vi "AI mnoz wartosci analogowe.vi"(6 "Mnozniki in":dbl[](array[numeric]), 7 "#cores (1)":i32=1, 8 "error in (no error)":errorcluster, 10 "Kanaly in":T1) -> (0 "error out":errorcluster, 2 "Kanaly out":T1, 5 "Niezgodnosc rozmiarow?":bool)   [LabVIEW 2013]
doc: "Mnoży wartości na aktywnych kanałach analogowych\nprzez mnożniki wyliczone z ustawien kart analogowych przystawki"
uses:
  Kontrolki/Przetwarzanie/Kanaly.ctl
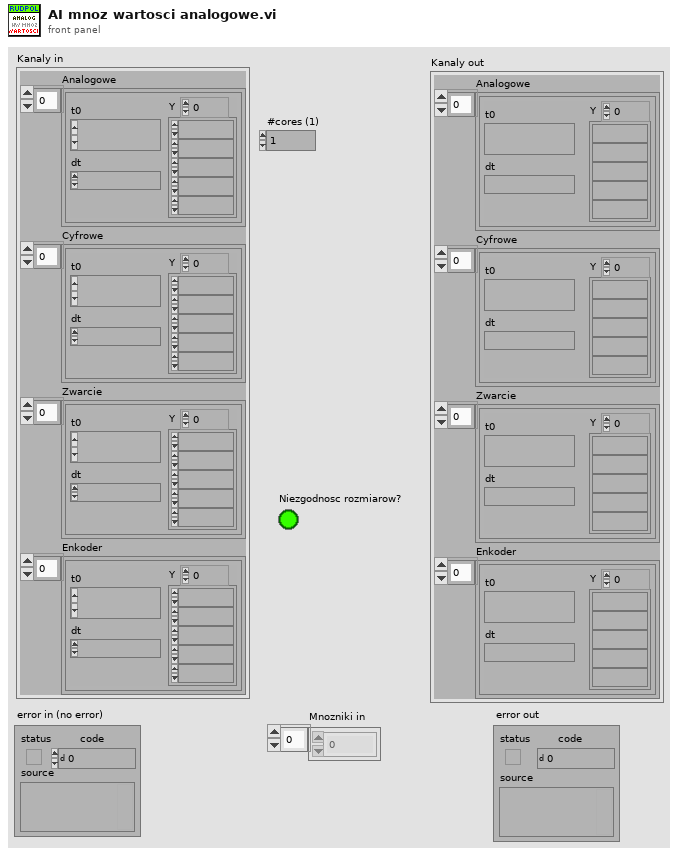
[diagram p1: front panel]
types:
  T1 = typedef "Kanaly.ctl" = cluster{"Analogowe":waveform(dbl)[], "Cyfrowe":waveform(dbl)[], "Zwarcie":waveform(dbl)[], "Enkoder":waveform(dbl)[]}
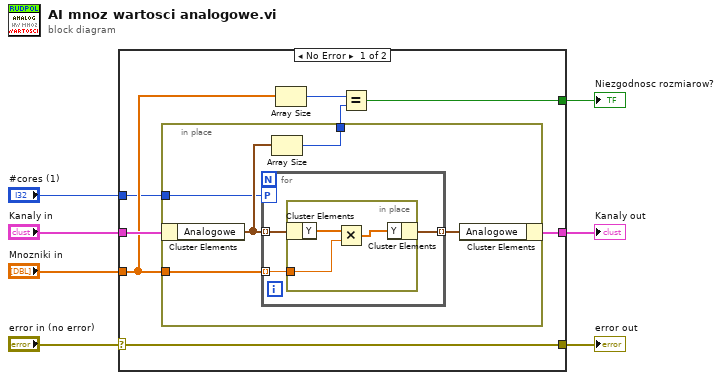
[diagram p0: block diagram]
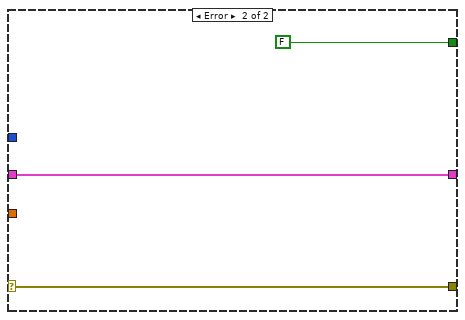
[diagram p2: hidden frame]
diagram:
  n1 = case shown="No Error" "error in (no error)" {
    selector: "error in (no error)" -> [w15 w29]
    tunnel: [w15 w29] -> w6
    tunnel: "Kanaly in" -> [w14 w28]
    tunnel: [w13 w28] -> w4
    tunnel: "Mnozniki in" -> [w12 _]
    tunnel: [w9 FALSE] -> w2
    tunnel: "#cores (1)" -> [w8 _]
    frame No Error {
      n2 = in-place {
        in-place-border: w12 -> [w20]
        in-place-border: [w18] -> w10
        in-place-border: w8 -> [w16]
        n3 = in-place-cluster #1(w14) -> ("Analogowe"=w19:waveform(dbl)[])
        n4 = for {
          tunnel: w19 -> [w23] mode=indexing
          tunnel: w20 -> [w22] mode=indexing
          tunnel: [w21] -> w17 mode=indexing
          workers-P: w16 -> [_]
          n5 = in-place {
            in-place-border: w22 -> [w25]
            n6 = in-place-cluster #2(w23) -> ("Y"=w26:dbl[])
            n7 = Multiply(x=w26, y=w25) -> (x*y=w24:dbl[])
            n8 = in-place-cluster #2("Y"=w24) -> (w21:waveform(dbl))
          }
        }
        n9 = Array Size(array=w19) -> (size(s)=w18:i32)
        n10 = in-place-cluster #1("Analogowe"=w17) -> (w13:T1)
      }
      n11 = Array Size(array=w12) -> (size(s)=w11:i32)
      n12 = Equal?(x=w11, y=w10) -> (x = y?=w9:bool)
    }
    frame Error {
    }
  }
  "error out" <- w6
  "Kanaly out" <- w4
  "Niezgodnosc rozmiarow?" <- w2
